vi "StartProcesses.vi"(8 "error in (no error)":errorcluster, 11 "SMO":refnum<class "SMO.lvclass">) -> (0 "error out":errorcluster, 3 "SMO out":refnum<class "SMO.lvclass">)   [LabVIEW 2019, in "SMO.lvclass"]
doc: "---------------------------------------------------------------\nJKI State Machine Objects™\nhttp://jki.net/state-machine-objects/\nCopyright (C) 2005-2015, JKI <info@jki.net>\nALL RIGHTS RESERVEDJKI State Machine Objects (SMO) 1.3.0.56\nJKI - JKI\nCopyright (c) 2017, JKI"
uses:
  SMO.lvclass
panel:
  # "For instructions on how to use the JKI State Machine Objects, examples and video tutorials, visit:\nhttp://jki.net/state-machine-objects/\n\nJKI State Machine Objects™\nhttp://jki.net/state-machine-objects/\nCopyright (C) 2005-2015, JKI <info@jki.net>\nALL RIGHTS RESERVED"
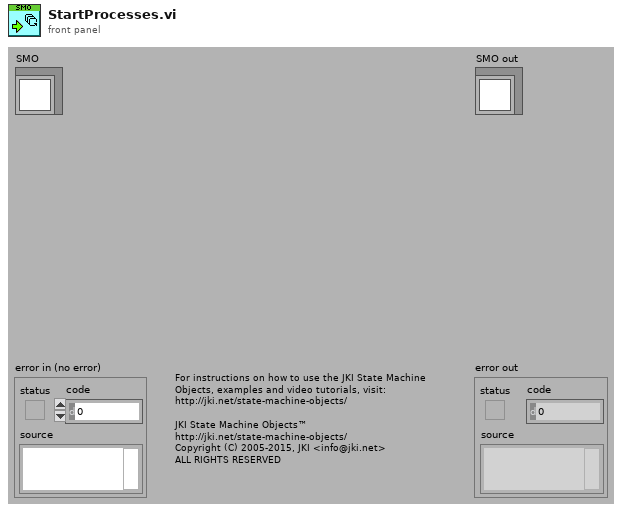
[diagram p1: front panel]
types:
  T1 = typedef "Attribute.StartupBehavior.lvclass/ProcessStartupBehavior.ctl" = enum16{"Immediate", "First Call", "Never"}
  T2 = typedef "SMO.lvclass/Public Events.ctl" = cluster{"Error":refnum<user-event>, "State":refnum<user-event>, "Reserve State":refnum<user-event>}
  T3 = typedef "SMO.lvclass/SMOState --Enum.ctl" = enum16{"unknown", "Created", "Started", "Stopped"}
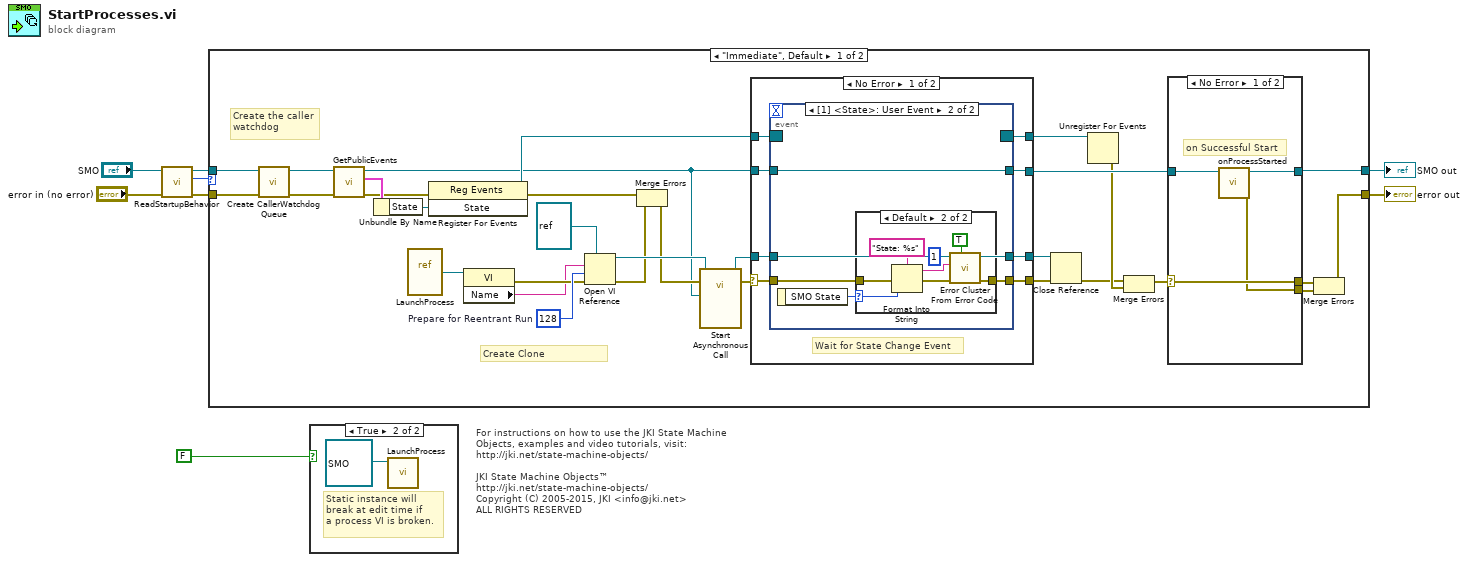
[diagram p0: block diagram]
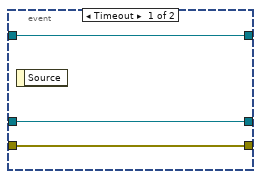
[diagram p2: hidden frame]
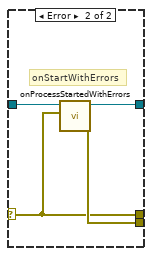
[diagram p5: hidden frame]
diagram:
  # "For instructions on how to use the JKI State Machine Objects, examples and video tutorials, visit:\nhttp://jki.net/state-machine-objects/\n\nJKI State Machine Objects™\nhttp://jki.net/state-machine-objects/\nCopyright (C) 2005-2015, JKI <info@jki.net>\nALL RIGHTS RESERVED"
  n1 = call "ReadStartupBehavior.vi"("error in (no error)"="error in (no error)", "SMO in"="SMO") -> ("error out"=w1:errorcluster, "Behavior"=w2:T1, "SMO out"=w4:refnum<class "SMO.lvclass">)  [unwired: 7 in]
  n2 = case shown="\"Immediate\", Default" w2 {
    tunnel: [w39 w78] -> w8
    tunnel: [w29 w77] -> w6
    tunnel: w4 -> [w14 w78]
    tunnel: w1 -> [w12 w77]
    frame "Immediate", Default {
      w38 = 128  # Prepare for Reentrant Run
      # "Create the caller\nwatchdog"
      # "Create Clone"
      n3 = call "Create CallerWatchdog Queue.vi"("error in (no error)"=w12, "SMO in"=w14) -> ("error out"=w11:errorcluster, "SMO out"=w13:refnum<class "SMO.lvclass">)  [unwired: 8 in]
      n4 = call "GetPublicEvents.vi"("error in (no error)"=w11, "SMO"=w13) -> ("error out"=w27:errorcluster, "Public Events"=w33:T2, "SMO out"=w10:refnum<class "SMO.lvclass">)  [unwired: 7 in]
      n5 = Unbundle By Name(w33) -> ("State"=w32:refnum<user-event>)
      n6 = vi-ref "LaunchProcess.vi"() -> (w35:refnum<vi>)
      n7 = register-events(error in=w27, w32) -> (reference out=w25:refnum<event-registration>, error out=w9:errorcluster)  [unwired: 1 in]
      n8 = property class="VI"(reference=w35) -> (error out=w37:errorcluster, "Name"=w36:string)  [unwired: 1 in, 1 out]
      n9 = Open VI Reference(type specifier VI Refnum (for type only)=refnum<vi> refnum ("reference out"), vi path=w36, options=w38, error in (no error)=w37) -> (vi reference=w34:refnum<vi>, error out=w24:errorcluster)  [unwired: 1 in, 1 out]
      n10 = Merge Errors(w9, w24) -> (w23:errorcluster)
      n11 = call-by-ref "Start Asynchronous Call"(reference=w34, error in=w23, "SMO Reference"=w10) -> (reference out=w22:refnum<vi>, error out=w26:errorcluster)  [unwired: 11 in]
      n12 = case shown="No Error" w26 {
        selector: w26 -> [w46 w66]
        tunnel: w10 -> [w44 w68]
        tunnel: [w43 w66] -> w18
        tunnel: [w45 w68] -> w31
        tunnel: w25 -> [w47 w67]
        tunnel: w22 -> [w40 w65]
        tunnel: [w42 w67] -> w20
        tunnel: [w41 w65] -> w17
        frame No Error {
          # "Wait for State Change Event"
          n13 = event shown="[1] <State>: User Event" {
            selector: w47 -> [_ _]
            dyn-events: [_ _] -> w42
            timeout: _ -> [_ _]
            tunnel: w46 -> [w49 w54]
            tunnel: [w50 w55] -> w45
            tunnel: w44 -> [w50 w55]
            tunnel: [w49 w53] -> w43
            tunnel: [w48 w51] -> w41
            tunnel: w40 -> [w48 w51]
            event Timeout {
              n14 = event-data() -> ()  [unwired: 1 in, 1 out]
            }
            event User Event {
              n15 = event-data() -> ("SMO State"=w52:T3)  [unwired: 1 in]
              n16 = case shown="Default" w52 {
                selector: w52 -> [_ w57]
                tunnel: w54 -> [w56 w60]
                tunnel: [w56 w58] -> w53
                frame "Started" {
                }
                frame Default {
                  n17 = Format Into String(format string="State: %s", error in=w60, w57) -> (resulting string=w63:string, error out=w59:errorcluster)  [unwired: 1 in]
                  n18 = call <vilib>:"Error Cluster From Error Code.vi"("show call chain? (False)"=TRUE, "error in (no error)"=w59, "error message (\"\")"=w63, "error code (0)"=1) -> ("error out"=w58:errorcluster)  [unwired: 5 in]
                }
              }
            }
          }
        }
        frame Error {
        }
      }
      n19 = Close Reference(reference=w17, error in (no error)=w18) -> (error out=w16:errorcluster)
      n20 = Unregister For Events(event registration refnum=w20) -> (error out=w19:errorcluster)  [unwired: 1 in]
      n21 = Merge Errors(w16, w19) -> (w21:errorcluster)
      n22 = case shown="No Error" w21 {
        selector: w21 -> [w70 w73]
        tunnel: w31 -> [w72 w76]
        tunnel: [w71 w75] -> w39
        tunnel: [w70 w73] -> w30
        tunnel: [w69 w74] -> w28
        frame No Error {
          # "on Successful Start"
          n23 = call-dynamic "onProcessStarted.vi"("SMO"=w72) -> ("error out"=w69:errorcluster, "SMO out"=w71:refnum<class "SMO.lvclass">)  [unwired: 9 in]
        }
        frame Error {
          # "onStartWithErrors"
          n24 = call-dynamic "onProcessStartedWithErrors.vi"("Start error"=w73, "SMO"=w76) -> ("error out"=w74:errorcluster, "SMO out"=w75:refnum<class "SMO.lvclass">)  [unwired: 8 in]
        }
      }
      n25 = Merge Errors(w30, w28) -> (w29:errorcluster)
    }
    frame "Never" {
    }
  }
  "error out" <- w6
  "SMO out" <- w8
  n26 = case shown="True" FALSE {
    frame False {
    }
    frame True {
      # "Static instance will\nbreak at edit time if\na process VI is broken."
      n27 = call "LaunchProcess.vi"("SMO Reference"=refnum<class "SMO.lvclass"> refnum ("JKI SMO.lvclass")) -> ()  [unwired: 11 in]
    }
  }
